vi "GetEntryWaveVoltageHigh.vi"(2 "Element":i16=1 min=1, 4 "error in (no error)":errorcluster, 5 "Return Parameter":u8(ring) items=["Value", "Minimum", "Maximum"], 6 "Channel":u16(ring) items=["Channel 1", "Channel 2", "Channel 3", "Channel 4", "Channel 5", "Channel 6", "Channel 7", "Channel 8"], 7 "VISA resource name":refnum<visa-resource-name>) -> (0 "error out":errorcluster, 1 "Voltage High (V)":dbl format="%#_16g", 3 "VISA resource name out":refnum<visa-resource-name>)   [LabVIEW 2020, in "Active Technologies AWG3000.lvlib"]
uses:
  Active Technologies AWG3000.lvlib
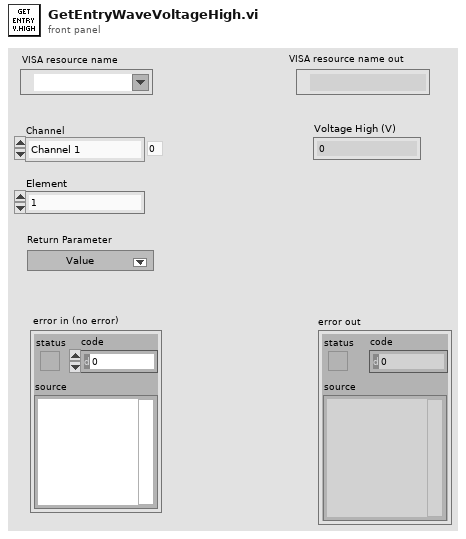
[diagram p1: front panel]
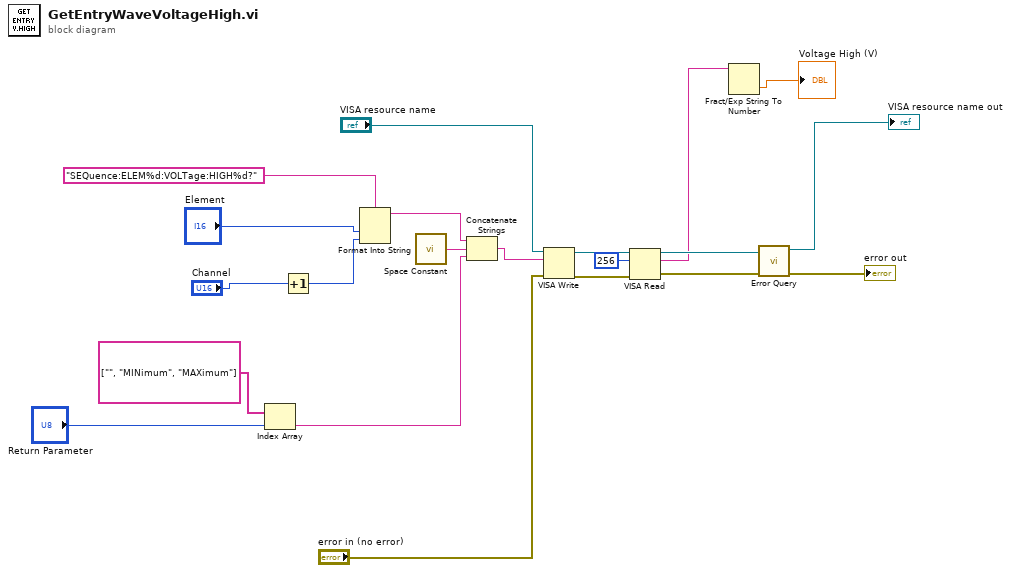
[diagram p0: block diagram]
diagram:
  n1 = Index Array(array=string[] ["", "MINimum", "MAXimum"], index="Return Parameter") -> (element=w7:string)
  n2 = Increment(x="Channel") -> (x+1=w4:u16)
  n3 = Format Into String(format string="SEQuence:ELEM%d:VOLTage:HIGH%d?" ("write buffer"), "Element", w4) -> (resulting string=w16:string)  [unwired: 2 in, 1 out]
  n4 = call <vilib>:"Space Constant.vi"() -> ("String"=w6:string)
  n5 = Concatenate Strings(w16, w6, w7) -> (w15:string)
  n6 = VISA Write(VISA resource name="VISA resource name", write buffer=w15, error in (no error)="error in (no error)") -> (VISA resource name out=w14:refnum<visa-resource-name>, error out=w13:errorcluster)  [unwired: 1 out]
  n7 = VISA Read(VISA resource name=w14, byte count=u32 256, error in (no error)=w13) -> (VISA resource name out=w11:refnum<visa-resource-name>, read buffer=w5:string, error out=w10:errorcluster)  [unwired: 1 out]
  n8 = Fract/Exp String To Number(string=w5) -> (number=→"Voltage High (V)":dbl)  [unwired: 3 in, 1 out]
  n9 = call "Error Query.vi"("error in (no error)"=w10, "VISA resource name"=w11) -> ("error out"=→"error out":errorcluster, "VISA resource name out"=→"VISA resource name out":refnum<visa-resource-name>)  [unwired: 6 in, 2 out]
